vi "time_gmtsec_weather.vi"(2 "Timezone Offset (Hrs)":i32=5, 3 "Timestamp":timestamp) -> (0 "Fractional Sec Since 12AM GMT":dbl, 1 "Sec Since 12AM GMT":u32)   [LabVIEW 2018]
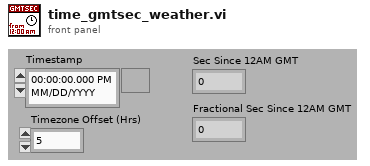
[diagram p1: front panel]
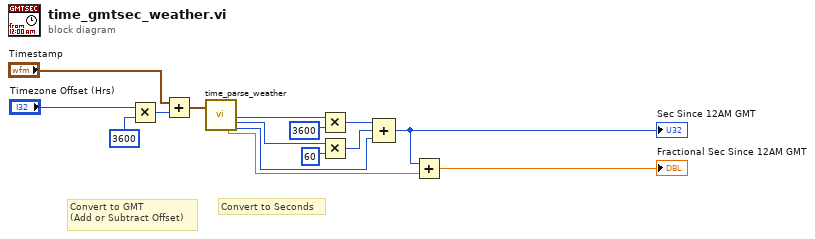
[diagram p0: block diagram]
diagram:
  # "Convert to Seconds"
  # "Convert to GMT\n(Add or Subtract Offset)"
  n1 = Multiply(x="Timezone Offset (Hrs)", y=3600) -> (x*y=w9:i32)
  n2 = Add(x="Timestamp", y=w9) -> (x+y=w11:timestamp)
  n3 = call "time_parse_weather.vi"("Current Time"=w11) -> ("Fractional Seconds"=w3:dbl, "Hour"=w15:u32, "Minutes"=w14:u32, "Seconds"=w6:u32)  [unwired: 12 in, 3 out]
  n4 = Multiply(x=w15, y=u32 3600) -> (x*y=w4:u32)
  n5 = Multiply(x=w14, y=u32 60) -> (x*y=w5:u32)
  n6 = Compound Arithmetic op=ADD(w4, w5, w6) -> (w1:u32)
  "Sec Since 12AM GMT" <- w1
  n7 = Add(x=w1, y=w3) -> (x+y=→"Fractional Sec Since 12AM GMT":dbl)
